vi "GetCtrlInfo.vi"(10 "Ctrl Label":string, 11 "UI Ref cluster":T2) -> (2 "Found":bool, 3 "Control out":refnum<vi>)   [LabVIEW 2018, in "UI_Library.lvlib" / "UI_Library.lvclass"]
doc: "Get Control info by name"
uses:
  UI_Library.lvclass
  <vilib>/Utility/Data Type/Type Definitions/Data Type.ctl
  <vilib>/Utility/Data Type/NI_Data Type.lvlib
  Controls/UI_RefCluster.ctl
  UI_Library.lvlib
panel:
  out "Type":T1
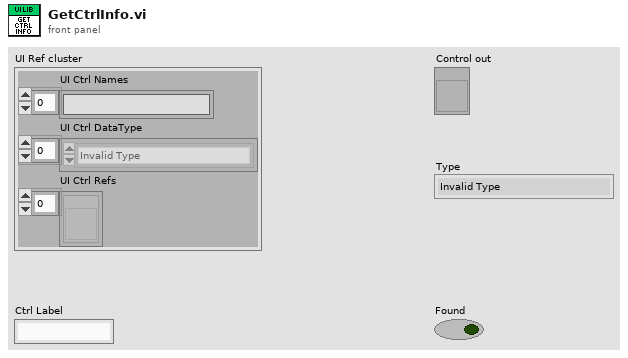
[diagram p1: front panel]
types:
  T1 = typedef "NI_Data Type.lvlib/Data Type.ctl" = enum8{"Invalid Type", "Void", "I8", "I16", "I32", "I64", "U8", "U16", "U32", "U64", "Single Float", "Double Float", "Extended Float", "Single Complex", "Double Complex", "Extended Complex", "Enum U8", "Enum U16", "Enum U32", "Enum U64", "Single Float With Unit", "Double Float With Unit", "Extended Float With Unit", "Single Complex with Unit", "Double Complex with Unit", "Extended Complex with Unit", "Boolean", "String", "Path", "Picture", "Tag", "Array", "Cluster", "Variant", "LV Variant", "Waveform", "Timestamp", "Digital Waveform", "Digital Data", "ExpressData", "Refnum", "External Data", "VI", "Poly VI", "LabVIEW Class Instance", "Fixed Point", "Set Collection", "Map Collection"}
  T2 = typedef "UI_Library.lvlib/UI_RefCluster.ctl" = cluster{"UI Ctrl Names":string[], "UI Ctrl DataType":T1[], "UI Ctrl Refs":refnum<vi>[]}
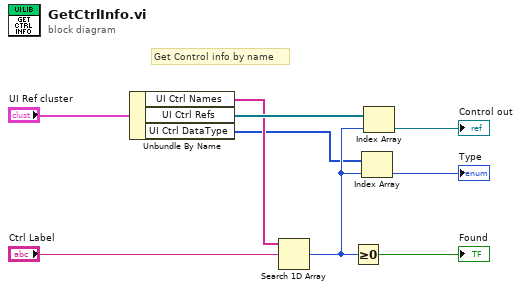
[diagram p0: block diagram]
diagram:
  # "Get Control info by name"
  n1 = Unbundle By Name("UI Ref cluster") -> ("UI Ctrl Names"=w4:string[], "UI Ctrl Refs"=w6:refnum<vi>[], "UI Ctrl DataType"=w2:T1[])
  n2 = Search 1D Array(1D array=w4, element="Ctrl Label") -> (index of element=w3:i32)  [unwired: 1 in]
  n3 = Greater Or Equal To 0?(x=w3) -> (x >= 0?=→"Found":bool)
  n4 = Index Array(array=w2, index=w3) -> (element=→"Type":T1)
  n5 = Index Array(array=w6, index=w3) -> (element=→"Control out":refnum<vi>)
